vi "FURBOLP.vi"() -> ()   [LabVIEW 2014]
panel:
  in  "Tab Control":enum32{"Login", "Main"}(tab)
  in  "login":bool
  in  "Password":string
  in  "Username":string
  out "Time Dispay":string
  out "Date":string
  out "Current set value":dbl format="%.1f"
  in  "Temp controller COM PORT":refnum<visa-resource-name>
  in  "Alarm set value":dbl format="%.1f"
  in  "Hour (24)":i8
  in  "Minute":i8
  in  "Day":i8
  in  "Month":i8
  in  "Alarm On":bool
  in  "Date On":bool
  in  "Set Value":bool
  in  "SV":dbl format="%.1f"
  out "PV value 2":dbl=1.0 format="%.1f"
  out "PV Value":dbl(slide) scale=0.0..120.0
  in  "?":bool
  # "Howdy Partner,\nWe don't take kindly to no snoopin' strangers in these parts. If you're going to be awantin' to use this here heater, then we're gonna need to see one of them username password contraptions first. \n                             (Username hint: Deep Red Woodland Clearing Mountain)\n                              (Password Hint: it's the last names of our PI's in abc order) \nSincerely,\nMr. Peltier \"the Oven\""
  # "TURBO CONTROLLER"
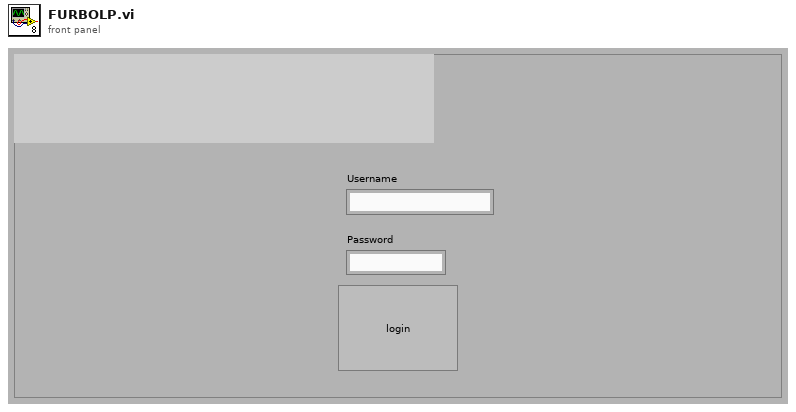
[diagram p1: front panel]
types:
  T1 = cluster{"Measurement":string, "Tags":string[][], "Fields":string[][]}
  T2 = cluster{"Measurement":string, "Tags":string[][], string[][]}
  T3 = typedef "imagedata.ctl" = cluster{"image type":i32, "image depth":i32, "image":u8[], "mask":u8[], "colors":u32[], "Rectangle":cluster{"left":i16, "top":i16, "right":i16, "bottom":i16}}
  T4 = typedef "LVRemotePanelConnectionsTypeDef.ctl" = cluster{"VI Name":string, "Remote":string, "UserName":string, "Port":i32, "Status":enum32{"Viewing", "Waiting For Control", "Controlling"}, "Create Time":timestamp, "Status Time":timestamp, "Control End Time":timestamp}[]
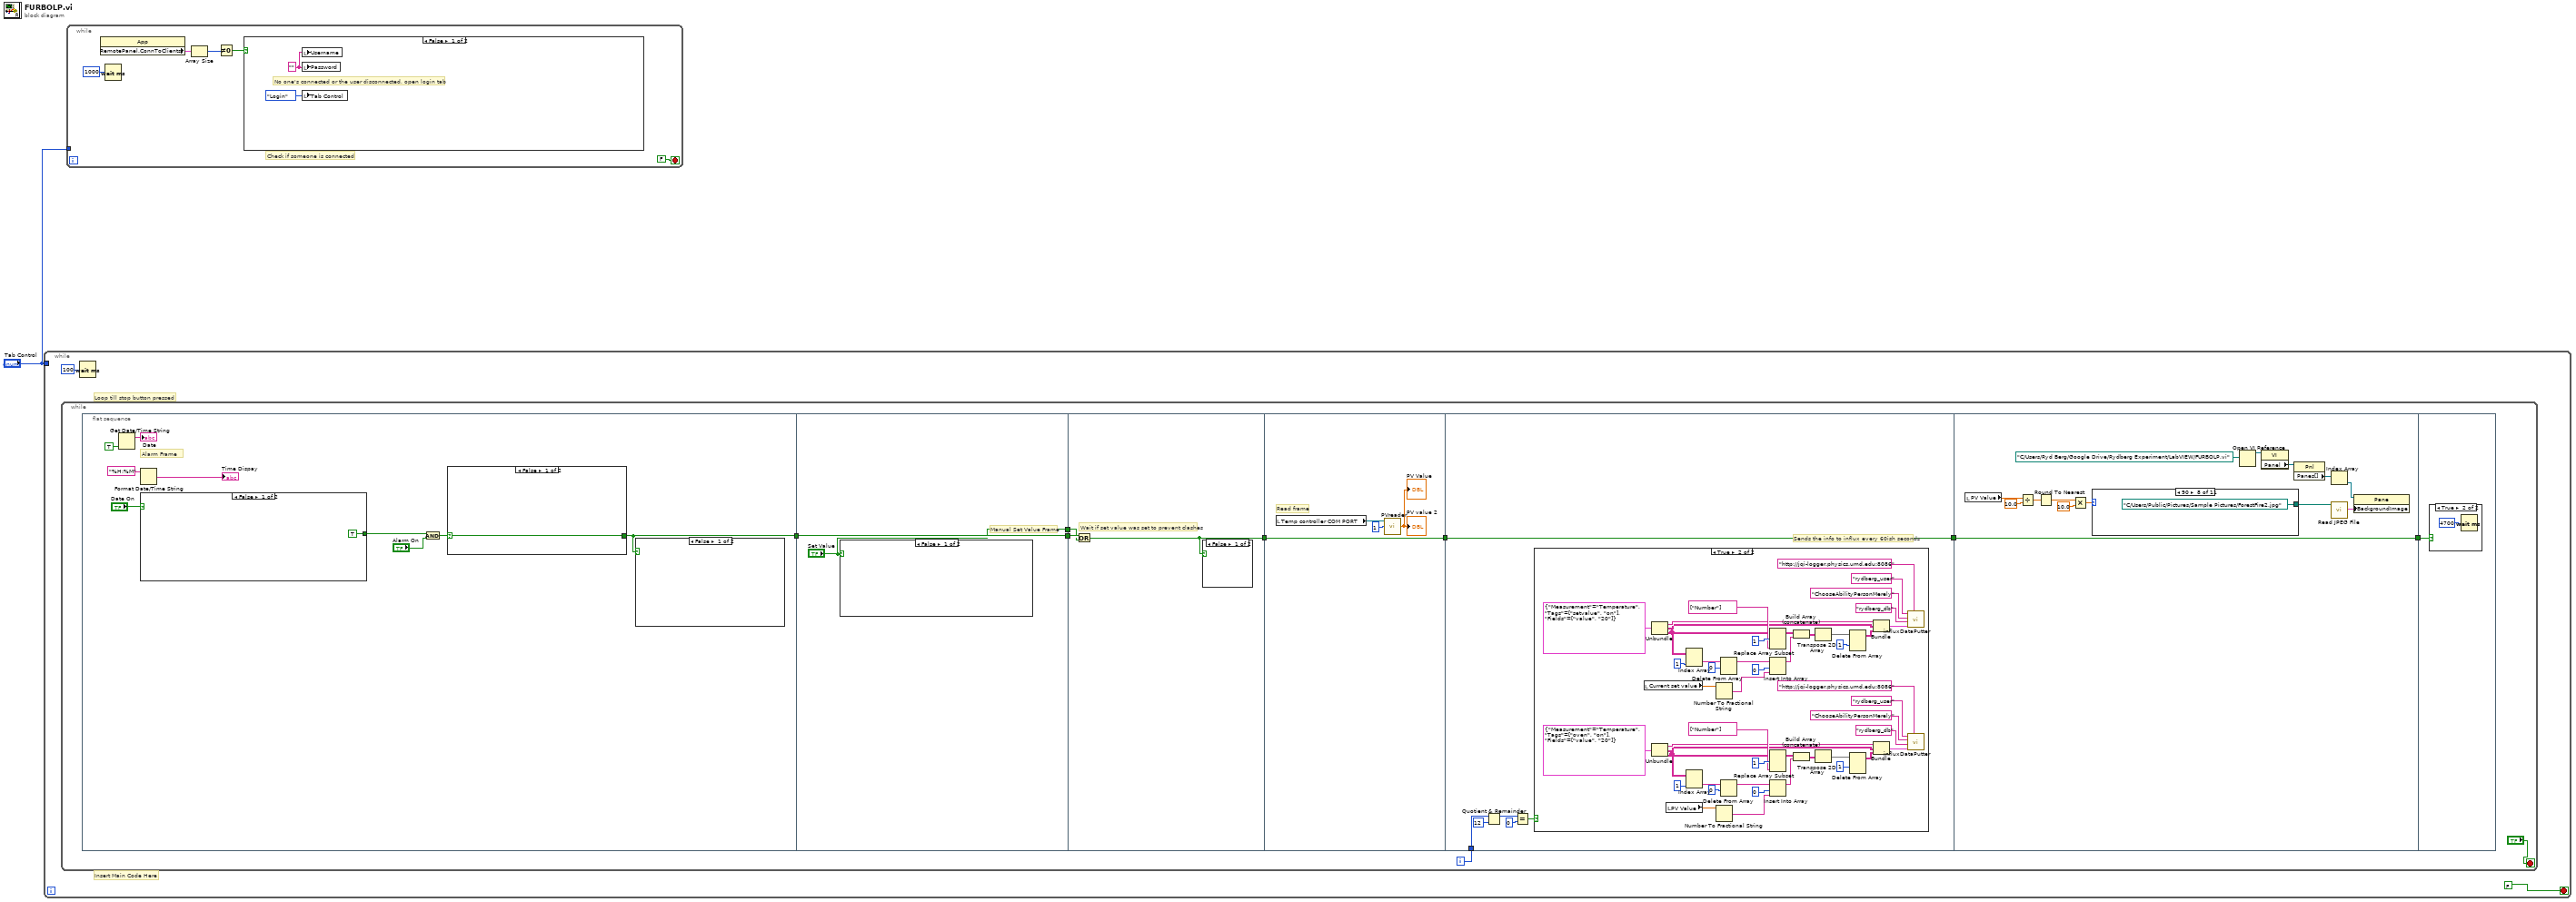
[diagram p0: block diagram]
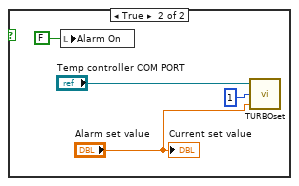
[diagram p2: hidden frame]
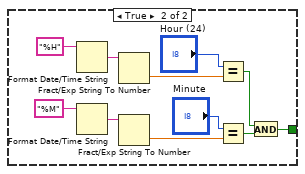
[diagram p3: hidden frame]
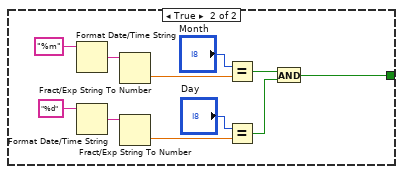
[diagram p4: hidden frame]
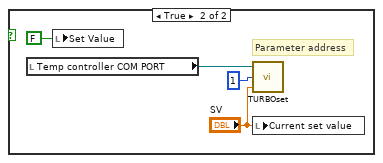
[diagram p5: hidden frame]
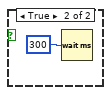
[diagram p6: hidden frame]
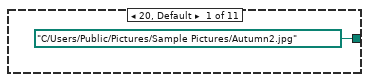
[diagram p8: hidden frame]
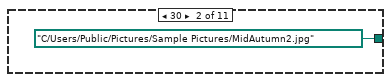
[diagram p9: hidden frame]
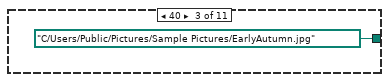
[diagram p10: hidden frame]
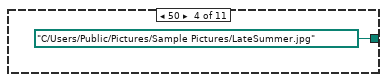
[diagram p11: hidden frame]
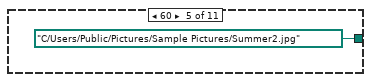
[diagram p12: hidden frame]
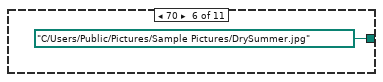
[diagram p13: hidden frame]
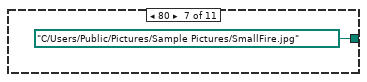
[diagram p14: hidden frame]
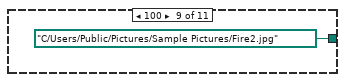
[diagram p15: hidden frame]
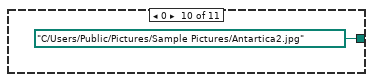
[diagram p16: hidden frame]
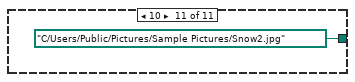
[diagram p17: hidden frame]
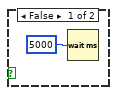
[diagram p18: hidden frame]
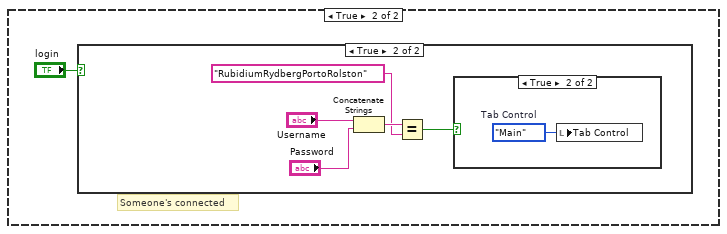
[diagram p19: hidden frame]
diagram:
  n1 = while {
    tunnel: "Tab Control" -> [_]
    stop <- FALSE stop-if-true
    # "Loop till stop button pressed"
    # "Insert Main Code Here"
    n2 = while {
      i -> [w7]
      stop <- "?" stop-if-true
      n3 = flat-sequence {
        tunnel: [w17] -> w11
        tunnel: [w51] -> w12
        tunnel: w11 -> [w51]
        tunnel: ["Set Value"] -> w10
        tunnel: w12 -> [w58]
        tunnel: w10 -> [w57]
        tunnel: [w56] -> w9
        tunnel: [w61] -> w8
        tunnel: w9 -> [w61]
        tunnel: w8 -> [w69]
        tunnel: [w69] -> w6
        tunnel: w7 -> [w68]
        tunnel: w6 -> [w131]
        tunnel: [w131] -> w5
        tunnel: w5 -> [w143]
        frame #0 {
          # "Alarm Frame"
          n4 = Get Date/Time String(want seconds? (F)=TRUE) -> (date string=→"Date":string)  [unwired: 2 in, 1 out]
          n5 = Format Date/Time String(time format string (%c)="%H:%M") -> (date/time string=→"Time Dispay":string)  [unwired: 2 in]
          n6 = case shown="False" "Date On" {
            tunnel: [TRUE w41] -> w20
            frame False {
            }
            frame True {
              n7 = Format Date/Time String(time format string (%c)="%m") -> (date/time string=w46:string)  [unwired: 2 in]
              n8 = Format Date/Time String(time format string (%c)="%d") -> (date/time string=w47:string)  [unwired: 2 in]
              n9 = Fract/Exp String To Number(string=w46) -> (number=w45:dbl)  [unwired: 3 in, 1 out]
              n10 = Fract/Exp String To Number(string=w47) -> (number=w44:dbl)  [unwired: 3 in, 1 out]
              n11 = Equal?(x="Month", y=w45) -> (x = y?=w42:bool)
              n12 = Equal?(x="Day", y=w44) -> (x = y?=w43:bool)
              n13 = And(x=w42, y=w43) -> (x .and. y?=w41:bool)
            }
          }
          n14 = And(x=w20, y="Alarm On") -> (x .and. y?=w18:bool)
          n15 = case shown="False" w18 {
            selector: w18 -> [w26 _]
            tunnel: [w26 w27] -> w17
            frame False {
            }
            frame True {
              n16 = Format Date/Time String(time format string (%c)="%H") -> (date/time string=w34:string)  [unwired: 2 in]
              n17 = Format Date/Time String(time format string (%c)="%M") -> (date/time string=w35:string)  [unwired: 2 in]
              n18 = Fract/Exp String To Number(string=w34) -> (number=w33:dbl)  [unwired: 3 in, 1 out]
              n19 = Fract/Exp String To Number(string=w35) -> (number=w32:dbl)  [unwired: 3 in, 1 out]
              n20 = Equal?(x="Hour (24)", y=w33) -> (x = y?=w30:bool)
              n21 = Equal?(x="Minute", y=w32) -> (x = y?=w31:bool)
              n22 = And(x=w30, y=w31) -> (x .and. y?=w27:bool)
            }
          }
          n23 = case shown="False" w17 {
            frame False {
            }
            frame True {
              n24 = local write "Alarm On"(FALSE ("Alarm On")) -> ()
              n25 = call "TURBOset.vi"("SV"="Alarm set value", "Device number"=i8 1, "VISA resource name"="Temp controller COM PORT") -> ()  [unwired: 1 out]
              "Current set value" <- "Alarm set value"
            }
          }
        }
        frame #1 {
          # "Manual Set Value Frame"
          n26 = case shown="False" "Set Value" {
            frame False {
            }
            frame True {
              # "Parameter address"
              n27 = local read "Temp controller COM PORT"() -> (w52:refnum<visa-resource-name>)
              n28 = local write "Set Value"(FALSE ("Value (Signaling)")) -> ()
              n29 = call "TURBOset.vi"("SV"="SV", "Device number"=i8 1, "VISA resource name"=w52) -> ()  [unwired: 1 out]
              n30 = local write "Current set value"("SV") -> ()
            }
          }
        }
        frame #2 {
          # "Wait if set value was set to prevent clashes"
          n31 = Or(x=w58, y=w57) -> (x .or. y?=w56:bool)
          n32 = case shown="False" w56 {
            frame False {
            }
            frame True {
              n33 = Wait (ms)(milliseconds to wait=u32 300) -> ()  [unwired: 1 out]
            }
          }
        }
        frame #3 {
          # "Read frame"
          n34 = local read "Temp controller COM PORT"() -> (w62:refnum<visa-resource-name>)
          n35 = call "PVreader.vi"("Device number"=i8 1, "VISA resource name"=w62) -> ("PV value"=→"PV Value" →"PV value 2":dbl)  [unwired: 1 in]
        }
        frame #4 {
          # "Sends the info to influx every 60ish seconds"
          n36 = Quotient & Remainder(x=w68, y=12) -> (x-y*floor(x/y)=w66:i32)  [unwired: 1 out]
          n37 = Equal?(x=w66, y=0) -> (x = y?=w64:bool)
          n38 = case shown="True" w64 {
            frame False {
            }
            frame True {
              n39 = local read "Current set value"() -> (w70:dbl)
              n40 = Unbundle(T1 {"Measurement"="Temperature", "Tags"=[["setvalue", "on"]], "Fields"=[["value", "20"]]} ("Data Cluster")) -> ("Measurement"=w77:string, "Tags"=w76:string[][], "Fields"=w88:string[][])
              n41 = Unbundle(T1 {"Measurement"="Temperature", "Tags"=[["oven", "on"]], "Fields"=[["value", "20"]]} ("Data Cluster")) -> ("Measurement"=w99:string, "Tags"=w98:string[][], "Fields"=w110:string[][])
              n42 = local read "PV Value"() -> (w71:dbl)
              n43 = Index Array(array=w88, index (col)=1) -> (element=w86:string[])  [unwired: 1 in]
              n44 = Index Array(array=w110, index (col)=1) -> (element=w108:string[])  [unwired: 1 in]
              n45 = Number To Fractional String(number=w70) -> (F-format string=w73:string)  [unwired: 3 in]
              n46 = Number To Fractional String(number=w71) -> (F-format string=w95:string)  [unwired: 3 in]
              n47 = Delete From Array(array=w86, length=0) -> (array with subset deleted=w84:string[])  [unwired: 1 in, 1 out]
              n48 = Delete From Array(array=w108, length=0) -> (array with subset deleted=w106:string[])  [unwired: 1 in, 1 out]
              n49 = Replace Array Subset(array=w88, new element=string[] ["Number"] ("new element/subarray"), index (row)=1 ("index")) -> (w81:string[][])  [unwired: 1 in]
              n50 = Insert Into Array(array=w84, index=0, new element=w73) -> (w82:string[])
              n51 = Replace Array Subset(array=w110, new element=string[] ["Number"] ("new element/subarray"), index (row)=1 ("index")) -> (w103:string[][])  [unwired: 1 in]
              n52 = Insert Into Array(array=w106, index=0, new element=w95) -> (w104:string[])
              n53 = Build Array (concatenate)(w81, w82) -> (w80:string[][])
              n54 = Build Array (concatenate)(w103, w104) -> (w102:string[][])
              n55 = Transpose 2D Array(2D array=w80) -> (transposed array=w79:string[][])
              n56 = Transpose 2D Array(2D array=w102) -> (transposed array=w101:string[][])
              n57 = Delete From Array(array=w79, index (row)=1) -> (array with subset deleted=w75:string[][])  [unwired: 2 in, 1 out]
              n58 = Delete From Array(array=w101, index (row)=1) -> (array with subset deleted=w97:string[][])  [unwired: 2 in, 1 out]
              n59 = Bundle("Measurement"=w77, "Tags"=w76, w75) -> (w74:T2)  [unwired: 1 in]
              n60 = Bundle("Measurement"=w99, "Tags"=w98, w97) -> (w96:T2)  [unwired: 1 in]
              n61 = call "influxDataPutter.vi"("Base URL"="http://jqi-logger.physics.umd.edu:8086", "Data Cluster"=w74, "Database Name"="rydberg_db", "Password"="ChooseAbilityPersonMerely", "Username"="rydberg_user") -> ()  [unwired: 4 in, 3 out]
              n62 = call "influxDataPutter.vi"("Base URL"="http://jqi-logger.physics.umd.edu:8086", "Data Cluster"=w96, "Database Name"="rydberg_db", "Password"="ChooseAbilityPersonMerely", "Username"="rydberg_user") -> ()  [unwired: 4 in, 3 out]
            }
          }
        }
        frame #5 {
          n63 = local read "PV Value"() -> (w124:dbl)
          n64 = Divide(x=w124, y=10.0) -> (x/y=w122:dbl)
          n65 = Round To Nearest(number=w122) -> (nearest integer value=w121:dbl)
          n66 = Multiply(x=w121, y=10.0) -> (x*y=w119:dbl)
          n67 = case shown="90" w119 {
            tunnel: [path "C:/Users/Public/Pictures/Sample Pictures/Autumn2.jpg" ("path to JPEG file") path "C:/Users/Public/Pictures/Sample Pictures/MidAutumn2.jpg" ("path to JPEG file") path "C:/Users/Public/Pictures/Sample Pictures/EarlyAutumn.jpg" ("path to JPEG file") path "C:/Users/Public/Pictures/Sample Pictures/LateSummer.jpg" ("path to JPEG file") path "C:/Users/Public/Pictures/Sample Pictures/Summer2.jpg" ("path to JPEG file") path "C:/Users/Public/Pictures/Sample Pictures/DrySummer.jpg" ("path to JPEG file") path "C:/Users/Public/Pictures/Sample Pictures/SmallFire.jpg" ("path to JPEG file") path "C:/Users/Public/Pictures/Sample Pictures/ForestFire2.jpg" ("path to JPEG file") path "C:/Users/Public/Pictures/Sample Pictures/Fire2.jpg" ("path to JPEG file") path "C:/Users/Public/Pictures/Sample Pictures/Antartica2.jpg" ("path to JPEG file") path "C:/Users/Public/Pictures/Sample Pictures/Snow2.jpg" ("path to JPEG file")] -> w118
            frame 20, Default {
            }
            frame 30 {
            }
            frame 40 {
            }
            frame 50 {
            }
            frame 60 {
            }
            frame 70 {
            }
            frame 80 {
            }
            frame 90 {
            }
            frame 100 {
            }
            frame 0 {
            }
            frame 10 {
            }
          }
          n68 = Open VI Reference(vi path=path "C:/Users/Ryd Berg/Google Drive/Rydberg Experiment/LabVIEW/FURBOLP.vi") -> (vi reference=w128:refnum<vi>)  [unwired: 1 in, 5 out]
          n69 = property class="VI"(reference=w128) -> ("Panel"=w130:refnum<vi>)  [unwired: 1 in, 2 out]
          n70 = property class="Pnl"(reference=w130) -> ("Panes[]"=w129:refnum<vi>[])  [unwired: 1 in, 2 out]
          n71 = Index Array(array=w129) -> (element=w127:refnum<vi>)  [unwired: 1 in]
          n72 = call <vilib>:"Read JPEG File.vi"("path to JPEG file"=w118) -> ("image data"=w126:T3)  [unwired: 1 in, 9 out]
          n73 = property class="Pane"(reference=w127, "BackgroundImage"=w126) -> ()  [unwired: 1 in, 2 out]
        }
        frame #6 {
          n74 = case shown="True" w143 {
            frame False {
              n75 = Wait (ms)(milliseconds to wait=u32 5000) -> ()  [unwired: 1 out]
            }
            frame True {
              n76 = Wait (ms)(milliseconds to wait=u32 4700) -> ()  [unwired: 1 out]
            }
          }
        }
      }
    }
    n77 = Wait (ms)(milliseconds to wait=u32 100) -> ()  [unwired: 1 out]
  }
  n78 = while {
    tunnel: "Tab Control" -> [_]
    stop <- FALSE stop-if-true
    # "Check if someone is connected"
    n79 = property class="App"() -> ("RemotePanel.ConnToClients"=w149:T4)  [unwired: 2 in, 2 out]
    n80 = Wait (ms)(milliseconds to wait=u32 1000) -> ()  [unwired: 1 out]
    n81 = Array Size(array=w149) -> (size(s)=w148:i32)
    n82 = Not Equal To 0?(x=w148) -> (x != 0?=w147:bool)
    n83 = case shown="False" w147 {
      frame False {
        w152 = ""
        # "No one's connected or the user disconnected, open login tab"
        n84 = local write "Username"(w152) -> ()
        n85 = local write "Password"(w152) -> ()
        n86 = local write "Tab Control"(enum32{"Login", "Main"}."Login" ("Tab Control")) -> ()
      }
      frame True {
        # "Someone's connected"
        n87 = case shown="True" "login" {
          frame False {
          }
          frame True {
            n88 = Concatenate Strings("Username", "Password") -> (w156:string)
            n89 = Equal?(x=w156, y="RubidiumRydbergPortoRolston") -> (x = y?=w154:bool)
            n90 = case shown="True" w154 {
              frame False {
              }
              frame True {
                w159 = enum32{"Login", "Main"}."Main"  # Tab Control
                n91 = local write "Tab Control"(w159) -> ()
              }
            }
          }
        }
      }
    }
  }
